vi "Perform Action.vi"(8 "error in (no error)":errorcluster, 10 "Input":variant, 11 "Sample PID Watervalve in":refnum<class "Sample PID Flow.lvclass">) -> (0 "error out":errorcluster, 2 "Output":variant, 3 "Sample PID Watervalve out":refnum<class "Sample PID Flow.lvclass">)   [LabVIEW 2023, in "Sample PID Flow.lvclass"]
uses:
  Sample PID Flow.lvclass
  D:/git/HAL/HAL GOOP4/Task/Task Base/Task Base.lvclass
  Task/Task Base/Task Base.lvclass/Task Base.ctl
  <vilib>/Utility/error.llb/Error Cluster From Error Code.vi
  <vilib>/addons/control/pid/pid.llb/PID (DBL).vi
  Sample PID Flow.lvclass/Sample PID Flow.ctl
  Task/Task Base/Task Base.lvclass
  Measure and Stimulus Subsystems/Measure and Stimulus Subsystems.lvclass
  <vilib>/addons/control/pid/NI_PID_pid.lvlib
  D:/git/HAL/HAL GOOP4/Tests/Sample Tasks/Sample PID Flow/Sample PID Flow.lvclass
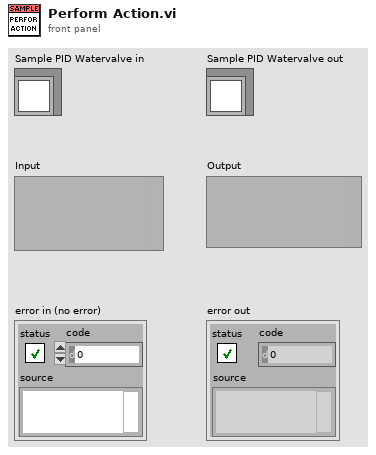
[diagram p1: front panel]
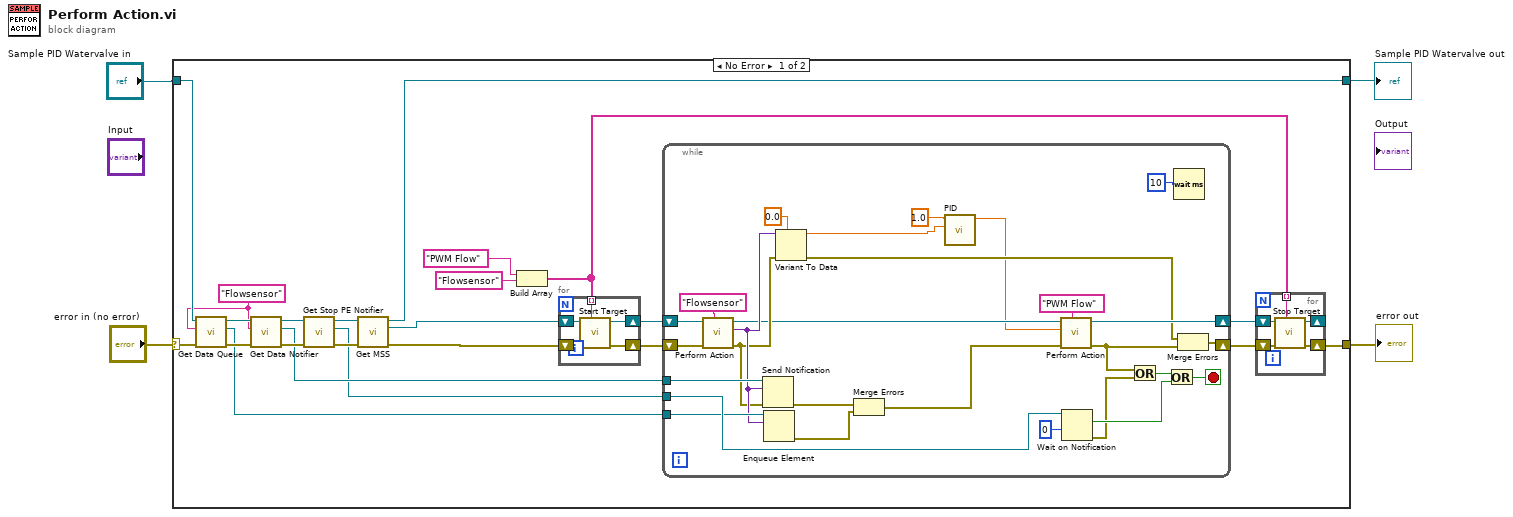
[diagram p0: block diagram]
diagram:
  n1 = case shown="No Error" "error in (no error)" {
    selector: "error in (no error)" -> [w24 w66]
    tunnel: [w20 w66] -> w1
    tunnel: [w11 w65] -> w2
    tunnel: "Sample PID Watervalve in" -> [w14 w65]
    frame No Error {
      w5 = "Flowsensor" ("Name")
      n2 = call "Get Data Queue.vi"("error in (no error)"=w24, "Target Name"=w5, "Task Base in"=w14) -> ("error out"=w15:errorcluster, "Data Queue"=w12:refnum<queue>, "Task Base out"=w13:refnum<class "Sample PID Flow.lvclass">)  [unwired: 6 in]
      n3 = call "Get Data Notifier.vi"("error in (no error)"=w15, "Target Name"=w5, "Task Base in"=w13) -> ("error out"=w19:errorcluster, "Data Notifier"=w10:refnum<notifier>, "Task Base out"=w8:refnum<class "Sample PID Flow.lvclass">)  [unwired: 6 in]
      n4 = call "Get Stop PE Notifier.vi"("error in (no error)"=w19, "Task Base in"=w8) -> ("error out"=w9:errorcluster, "Stop PE"=w6:refnum<notifier>, "Task Base out"=w7:refnum<class "Sample PID Flow.lvclass">)  [unwired: 7 in]
      n5 = call "Get MSS.vi"("error in (no error)"=w9, "Task Base in"=w7) -> ("error out"=w23:errorcluster, "MSS"=w22:refnum<class "Measure and Stimulus Subsystems.lvclass">, "Task Base in"=w11:refnum<class "Sample PID Flow.lvclass">)  [unwired: 7 in]
      n6 = Build Array("PWM Flow" ("Target Ident"), "Flowsensor" ("Target Identifier")) -> (w16:string[])
      n7 = for {
        shift-right: [w32] -> w27
        shift-left: w23 -> [w30]
        shift-right: [w31] -> w26
        shift-left: w22 -> [w29]
        tunnel: w16 -> [w28] mode=indexing
        n8 = call "Start Target.vi"("Target Ident"=w28, "Error In"=w30, "reference in"=w29) -> ("Error Out"=w32:errorcluster, "reference out"=w31:refnum<class "Measure and Stimulus Subsystems.lvclass">)  [unwired: 7 in]
      }
      n9 = while {
        shift-right: [w51] -> w25
        shift-left: w27 -> [w55]
        shift-right: [w57] -> w21
        shift-left: w26 -> [w54]
        tunnel: w6 -> [w45]
        tunnel: w10 -> [w46]
        tunnel: w12 -> [w41]
        stop <- w49 stop-if-true
        n10 = call "Perform Action.vi"("Target Ident"="Flowsensor" ("Target Identifier"), "Error In"=w55, "reference in"=w54) -> ("Error Out"=w35:errorcluster, "Output"=w36:variant, "reference out"=w34:refnum<class "Measure and Stimulus Subsystems.lvclass">)  [unwired: 6 in]
        n11 = Send Notification(notification=w36, notifier=w46, error in (no error)=w35) -> (error out=w38:errorcluster)  [unwired: 1 out]
        n12 = Enqueue Element(queue=w41, element=w36) -> (error out=w40:errorcluster)  [unwired: 2 in, 2 out]
        n13 = Variant To Data(error in=w35, type=0.0, Variant=w36) -> (data=w52:dbl, error out=w50:errorcluster)
        n14 = Merge Errors(w38, w40) -> (w39:errorcluster)
        n15 = call-poly <vilib>:"PID.vi"("process variable"=w52, "setpoint"=1.0) -> ("output"=w33:dbl)  [unwired: 8 in, 1 out]
        n16 = call "Perform Action.vi"("Target Ident"="PWM Flow", "Error In"=w39, "Input"=w33, "reference in"=w34) -> ("Error Out"=w42:errorcluster, "reference out"=w57:refnum<class "Measure and Stimulus Subsystems.lvclass">)  [unwired: 5 in, 1 out]
        n17 = Wait on Notification(notifier=w45, timeout in ms (-1)=0) -> (notification=w47:bool, error out=w44:errorcluster)  [unwired: 2 in, 2 out]
        n18 = Or(x=w42, y=w44) -> (x .or. y?=w43:bool)
        n19 = Or(x=w43, y=w47) -> (x .or. y?=w49:bool)
        n20 = Wait (ms)(milliseconds to wait=u32 10) -> ()  [unwired: 1 out]
        n21 = Merge Errors(w50, w42) -> (w51:errorcluster)
      }
      n22 = for {
        shift-right: [w62] -> w20
        shift-left: w25 -> [w64]
        tunnel: w16 -> [w61] mode=indexing
        shift-right: [w60] -> _
        shift-left: w21 -> [w63]
        n23 = call "Stop Target.vi"("Target Ident"=w61, "Error In"=w64, "reference in"=w63) -> ("Error Out"=w62:errorcluster, "reference out"=w60:refnum<class "Measure and Stimulus Subsystems.lvclass">)  [unwired: 7 in]
      }
    }
    frame Error {
    }
  }
  "error out" <- w1
  "Sample PID Watervalve out" <- w2
